vi "sumLinesIntoVolume.vi"(6 "calc ff/fb":bool, 7 "tracking":bool, 8 "error in (no error)":errorcluster, 9 "xyz order":bool, 10 "volumes to assemble":T2[](array[typedef])) -> (0 "error out":errorcluster, 1 "lines inserted":i32, 2 "volumes to send":cluster{"volume info":T1, u32[]}[](array[cluster]))   [LabVIEW 2010]
uses:
  volume_with_lines.ctl
  volume_info.ctl
  line_info.ctl
  get write location linear fit.vi
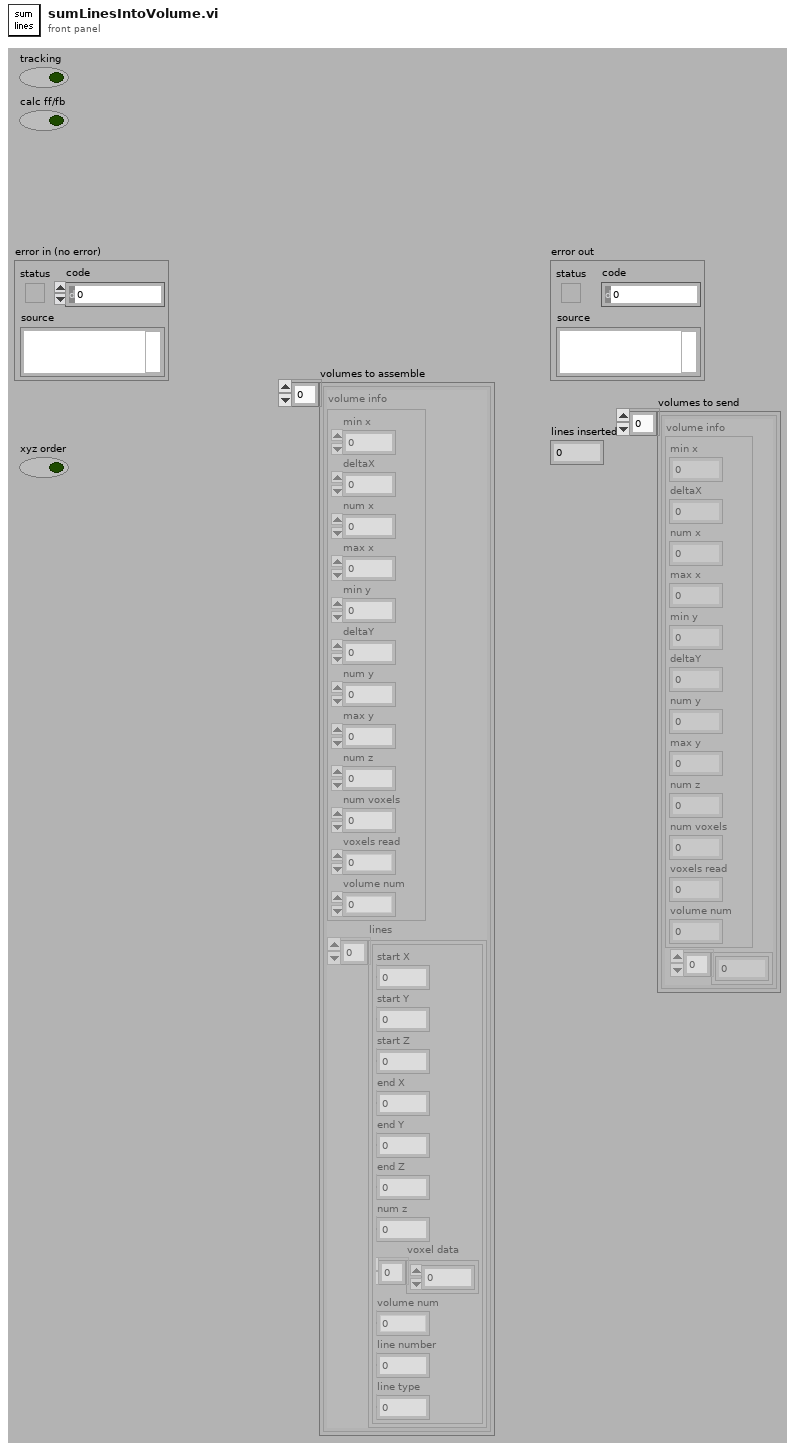
[diagram p1: front panel]
types:
  T1 = typedef "volume_info.ctl" = cluster{"min x":i16, "deltaX":dbl, "num x":u32, "max x":i16, "min y":i16, "deltaY":dbl, "num y":u32, "max y":i16, "num z":u32, "num voxels":u32, "voxels read":u32, "volume num":u32}
  T2 = typedef "volume_with_lines.ctl" = cluster{"volume info":T1, "lines":T3[]}
  T3 = typedef "line_info.ctl" = cluster{"start X":i16, "start Y":i16, "start Z":i16, "end X":i16, "end Y":i16, "end Z":i16, "num z":u8, "voxel data":u32[], "volume num":u32, "line number":u16, "line type":u16}
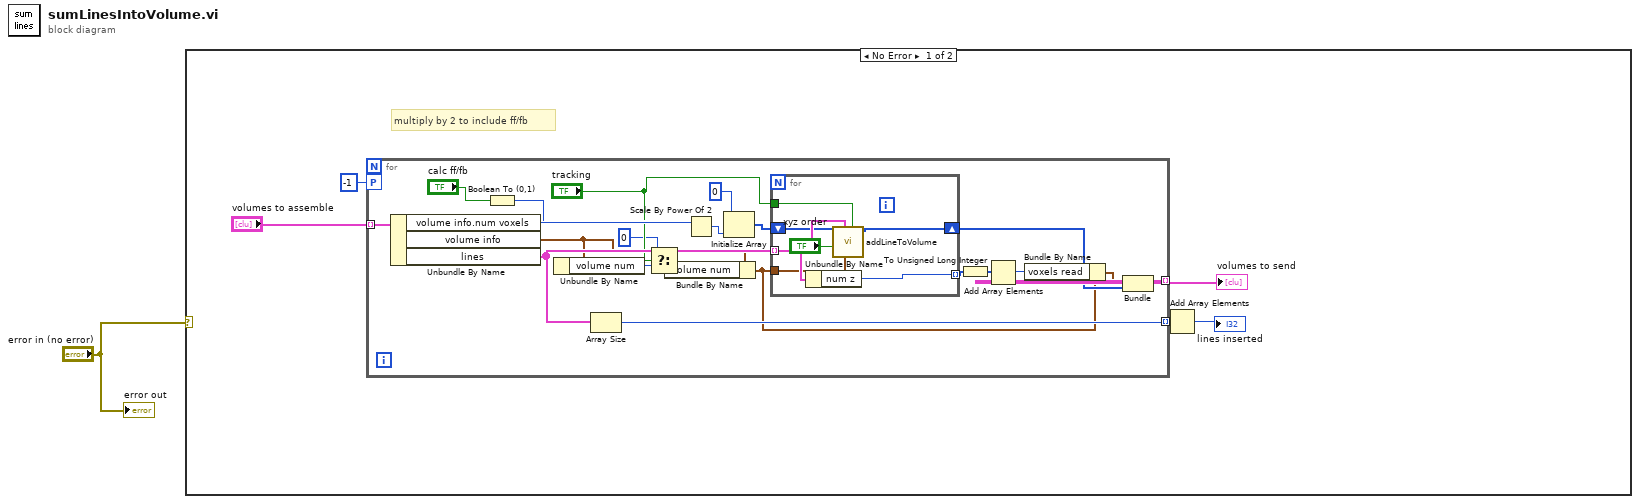
[diagram p0: block diagram]
diagram:
  n1 = case shown="No Error" "error in (no error)" {
    frame No Error {
      # "multiply by 2 to include ff/fb"
      n2 = for {
        tunnel: "volumes to assemble" -> [w27] mode=indexing
        tunnel: [w18] -> w5 mode=indexing
        workers-P: -1 -> [_]
        tunnel: [w15] -> w4 mode=indexing
        n3 = Unbundle By Name(w27) -> ("volume info.num voxels"=w26:u32, "volume info"=w12:T1, "lines"=w16:T3[])
        n4 = Boolean To (0,1)(Boolean="calc ff/fb") -> (0, 1=w14:i16)
        n5 = Unbundle By Name(w12) -> ("volume num"=w10:u32)
        n6 = Array Size(array=w16) -> (size(s)=w15:i32)
        n7 = Select(t=u32 0, s="tracking", f=w10) -> (s? t:f=w11:u32)
        n8 = Bundle By Name(cluster=w12, "volume num"=w11) -> (w7:T1)
        n9 = Scale By Power Of 2(n=w14, x=w26) -> (x*2^n=w25:u32)
        n10 = Initialize Array(u32 0, w25) -> (w23:u32[])
        n11 = for {
          tunnel: w7 -> [w32]
          tunnel: w16 -> [w33] mode=indexing
          shift-right: [w30] -> w19
          shift-left: w23 -> [w31]
          tunnel: [w34] -> w22 mode=indexing
          tunnel: "tracking" -> [w28]
          n12 = Unbundle By Name(w33) -> ("num z"=w34:u8)
          n13 = call "addLineToVolume.vi"("tracking"=w28, "current volume"=w32, "line"=w33, "xyz order"="xyz order", "volume buffer"=w31) -> ("volume buffer out"=w30:u32[])  [unwired: 5 in, 1 out]
        }
        n14 = To Unsigned Long Integer(number=w22) -> (unsigned 32bit integer=w17:u32[])
        n15 = Add Array Elements(numeric array=w17) -> (sum=w21:u32)
        n16 = Bundle By Name(cluster=w7, "voxels read"=w21) -> (w20:T1)
        n17 = Bundle("volume info"=w20, w19) -> (w18:cluster{"volume info":T1, u32[]})  [unwired: 1 in]
      }
      "volumes to send" <- w5
      n18 = Add Array Elements(numeric array=w4) -> (sum=→"lines inserted":i32)
    }
    frame Error {
    }
  }
  "error out" <- "error in (no error)"
